vi "id参数转换.vi"(11 "id":u16) -> (3 "table输出":string, 5 "数组资源索引":i32)   [LabVIEW 2016, in "斯坦道总氮V2.lvlib"]
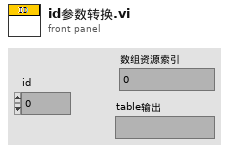
[diagram p1: front panel]
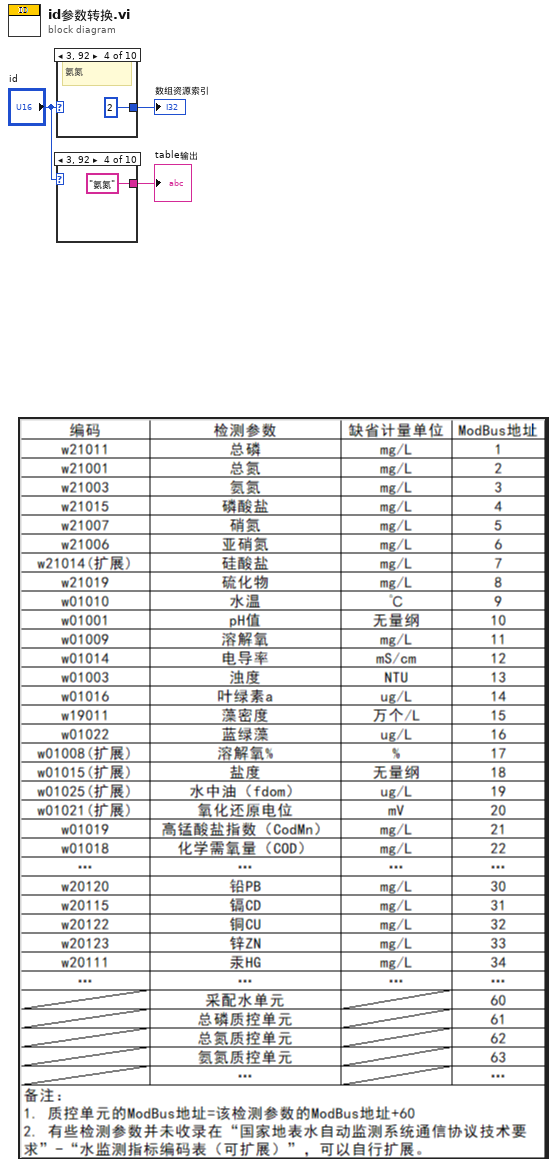
[diagram p0: block diagram]
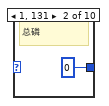
[diagram p3: hidden frame]
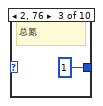
[diagram p4: hidden frame]
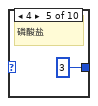
[diagram p5: hidden frame]
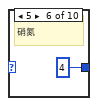
[diagram p6: hidden frame]
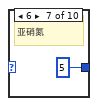
[diagram p7: hidden frame]
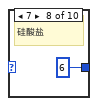
[diagram p8: hidden frame]
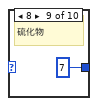
[diagram p9: hidden frame]
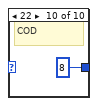
[diagram p10: hidden frame]
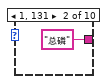
[diagram p12: hidden frame]
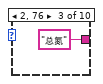
[diagram p13: hidden frame]
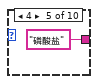
[diagram p14: hidden frame]
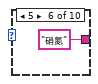
[diagram p15: hidden frame]
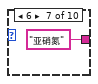
[diagram p16: hidden frame]
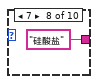
[diagram p17: hidden frame]
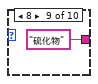
[diagram p18: hidden frame]
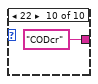
[diagram p19: hidden frame]
diagram:
  n1 = case shown="3, 92" "id" {
    selector: "id" -> [w4 _ _ _ _ _ _ _ _ _]
    tunnel: [w4 0 1 2 3 4 5 6 7 8] -> w1
    frame Default {
    }
    frame 1, 131 {
      # "总磷"
    }
    frame 2, 76 {
      # "总氮"
    }
    frame 3, 92 {
      # "氨氮"
    }
    frame 4 {
      # "磷酸盐"
    }
    frame 5 {
      # "硝氮"
    }
    frame 6 {
      # "亚硝氮"
    }
    frame 7 {
      # "硅酸盐"
    }
    frame 8 {
      # "硫化物"
    }
    frame 22 {
      # "COD"
    }
  }
  "数组资源索引" <- w1
  n2 = case shown="3, 92" "id" {
    tunnel: [_ "总磷" ("table输入") "总氮" ("table输入") "氨氮" ("table输入") "磷酸盐" ("table输入") "硝氮" ("table输入") "亚硝氮" ("table输入") "硅酸盐" ("table输入") "硫化物" ("table输入") "CODcr" ("table输入")] -> w3
    frame 0, Default {
    }
    frame 1, 131 {
    }
    frame 2, 76 {
    }
    frame 3, 92 {
    }
    frame 4 {
    }
    frame 5 {
    }
    frame 6 {
    }
    frame 7 {
    }
    frame 8 {
    }
    frame 22 {
    }
  }
  "table输出" <- w3
